vi "SET_START_STOP_MEASURE_FW.vi"(7 "LabVIEW Web Service Request":refnum<class "Web Request.lvclass">, 10 "TRIGGER":bool=TRUE, 11 "DEVICE_SN":string) -> (3 "Response":T1)   [LabVIEW 2015]
uses:
  <vilib>/wsapi/Web Request.lvclass
  Share Data/uPower_kit.ctl
panel:
  # "Use the Web Service Request input terminal to call the VIs on the Web Services palette. Do not remove it from the connector pane unless you don't need access to the palette."
  # "Each additional control wired to the connector pane will be available as an input in the URL. To include an indicator in terminal-mode output (the default setting), it must also be wired to the connector pane."
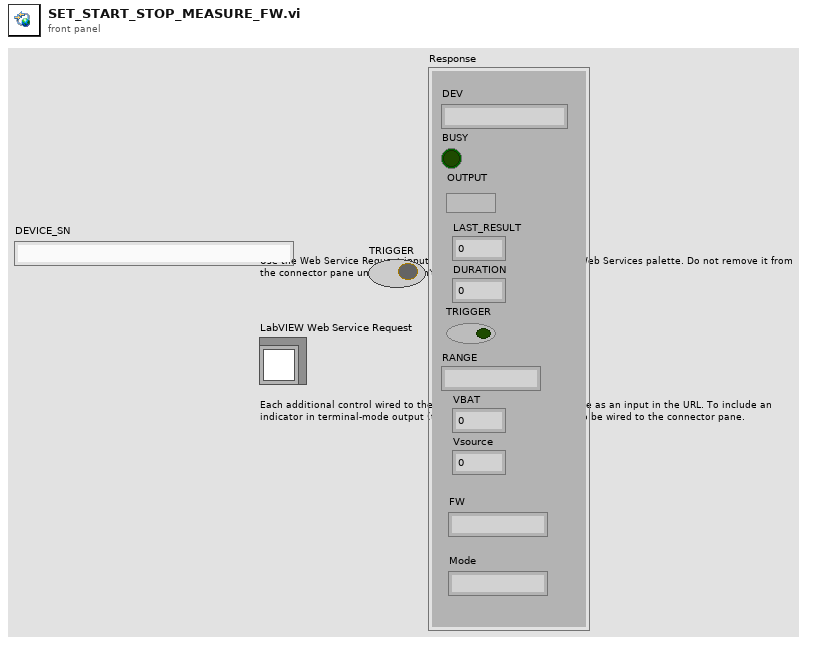
[diagram p1: front panel]
types:
  T1 = typedef "uPower_kit.ctl" = cluster{"DEV":string, "BUSY":bool, "VBAT":dbl, "OUTPUT":bool, "LAST_RESULT":dbl, "DURATION":u16, "TRIGGER":bool, "RANGE":string, "Vsource":dbl, "FW":string, "Mode":string}
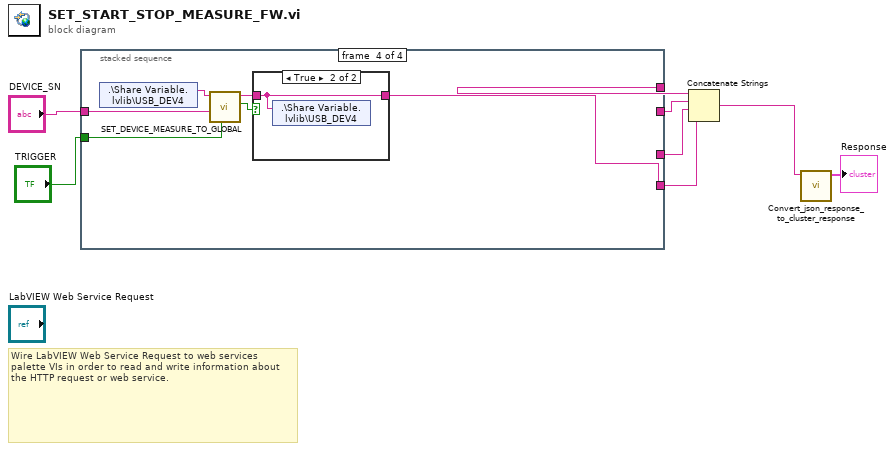
[diagram p0: block diagram]
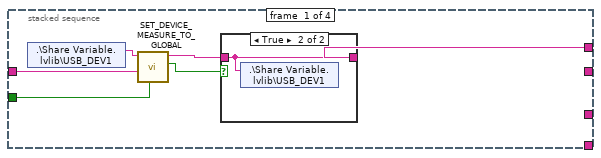
[diagram p2: hidden frame]
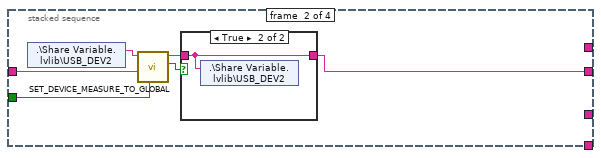
[diagram p4: hidden frame]
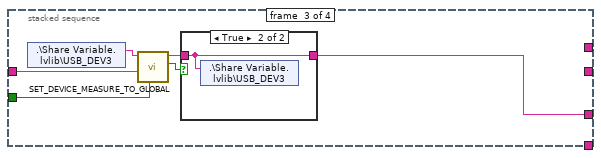
[diagram p6: hidden frame]
diagram:
  # "Wire LabVIEW Web Service Request to web services palette VIs in order to read and write information about the HTTP request or web service."
  n1 = stacked-sequence {
    tunnel: "DEVICE_SN" -> [w13 w20 w27 w34]
    tunnel: "TRIGGER" -> [w12 w19 w26 w33]
    tunnel: [w9 _ _ _] -> w6
    tunnel: [_ w16 _ _] -> w5
    tunnel: [_ _ w23 _] -> w2
    tunnel: [_ _ _ w30] -> w1
    frame #0 {
      n2 = shared-variable ".\\Share Variable.lvlib\\USB_DEV1"() -> (w14:string)  [unwired: 1 in, 1 out]
      n3 = call "SET_DEVICE_MEASURE_TO_GLOBAL.vi"("TRIGGER"=w12, "DEVICE in"=w13, "USB_DEV"=w14) -> ("DEVICE? 2"=w11:bool, "JSON string response 2"=w10:string)  [unwired: 7 in]
      n4 = case shown="True" w11 {
        tunnel: w10 -> [_ w15]
        tunnel: [_ w15] -> w9
        frame False {
        }
        frame True {
          n5 = shared-variable ".\\Share Variable.lvlib\\USB_DEV1"(w15) -> ()  [unwired: 1 in, 1 out]
        }
      }
    }
    frame #1 {
      n6 = shared-variable ".\\Share Variable.lvlib\\USB_DEV2"() -> (w21:string)  [unwired: 1 in, 1 out]
      n7 = call "SET_DEVICE_MEASURE_TO_GLOBAL.vi"("TRIGGER"=w19, "DEVICE in"=w20, "USB_DEV"=w21) -> ("DEVICE? 2"=w18:bool, "JSON string response 2"=w17:string)  [unwired: 7 in]
      n8 = case shown="True" w18 {
        tunnel: w17 -> [_ w22]
        tunnel: [_ w22] -> w16
        frame False {
        }
        frame True {
          n9 = shared-variable ".\\Share Variable.lvlib\\USB_DEV2"(w22) -> ()  [unwired: 1 in, 1 out]
        }
      }
    }
    frame #2 {
      n10 = shared-variable ".\\Share Variable.lvlib\\USB_DEV3"() -> (w28:string)  [unwired: 1 in, 1 out]
      n11 = call "SET_DEVICE_MEASURE_TO_GLOBAL.vi"("TRIGGER"=w26, "DEVICE in"=w27, "USB_DEV"=w28) -> ("DEVICE? 2"=w25:bool, "JSON string response 2"=w24:string)  [unwired: 7 in]
      n12 = case shown="True" w25 {
        tunnel: w24 -> [_ w29]
        tunnel: [_ w29] -> w23
        frame False {
        }
        frame True {
          n13 = shared-variable ".\\Share Variable.lvlib\\USB_DEV3"(w29) -> ()  [unwired: 1 in, 1 out]
        }
      }
    }
    frame #3 {
      n14 = shared-variable ".\\Share Variable.lvlib\\USB_DEV4"() -> (w35:string)  [unwired: 1 in, 1 out]
      n15 = call "SET_DEVICE_MEASURE_TO_GLOBAL.vi"("TRIGGER"=w33, "DEVICE in"=w34, "USB_DEV"=w35) -> ("DEVICE? 2"=w32:bool, "JSON string response 2"=w31:string)  [unwired: 7 in]
      n16 = case shown="True" w32 {
        tunnel: w31 -> [_ w36]
        tunnel: [_ w36] -> w30
        frame False {
        }
        frame True {
          n17 = shared-variable ".\\Share Variable.lvlib\\USB_DEV4"(w36) -> ()  [unwired: 1 in, 1 out]
        }
      }
    }
  }
  n18 = Concatenate Strings(w6, w5, w2, w1) -> (w4:string)
  n19 = call "Convert_json_response_to_cluster_response.vi"("Json_Response_in"=w4) -> ("Response"=→"Response":T1)  [unwired: 10 in]
